vi "ReadMVC.vi"(9 "Max Time (s)":dbl=10.0, 11 "MVC Path":path) -> (1 "MVCpos":i32[](array[numeric]), 2 "MVCvalue":dbl[](array[numeric]), 3 "Muscles":string[](array[string]))   [LabVIEW 2015]
uses:
  EMG/EMG.lvclass
panel:
  out "Waveform Graph":dbl[][](graph)
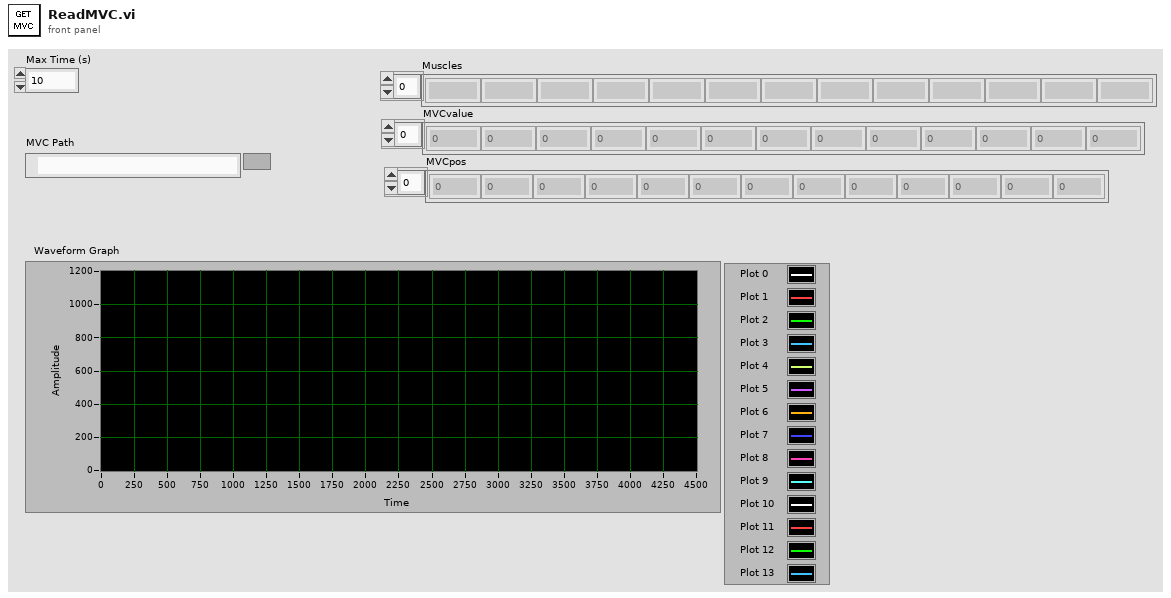
[diagram p1: front panel]
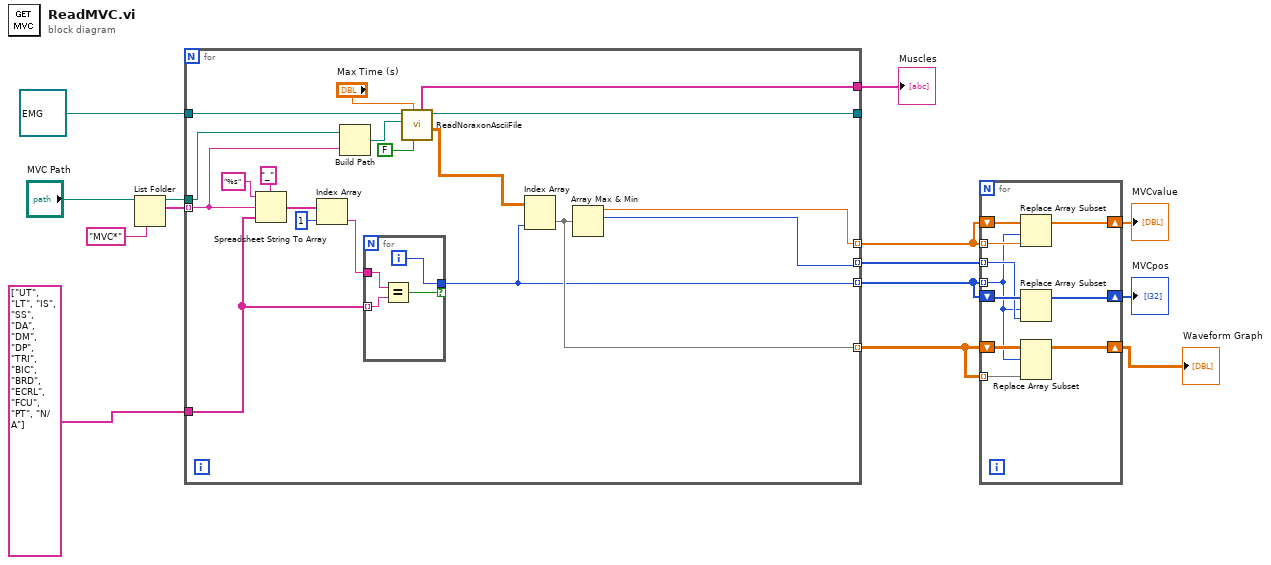
[diagram p0: block diagram]
diagram:
  n1 = List Folder(path="MVC Path", pattern="MVC*") -> (path out=w11:path, filenames=w12:string[])  [unwired: 2 in, 2 out]
  n2 = for {
    tunnel: w12 -> [w28] mode=indexing
    tunnel: w11 -> [w27]
    tunnel: string[] ["UT", "LT", "IS", "SS", "DA", "DM", "DP", "TRI", "BIC", "BRD", "ECRL", "FCU", "PT", "N/A"] -> [w26]
    tunnel: refnum<class "EMG.lvclass"> refnum ("EMG.lvclass") -> [w30]
    tunnel: [w24] -> _
    tunnel: [w15] -> w1
    tunnel: [w23] -> w4 mode=indexing
    tunnel: [w22] -> w8 mode=indexing
    tunnel: [w17] -> w5 mode=indexing
    tunnel: [w20] -> w2 mode=indexing
    n3 = Spreadsheet String To Array(delimiter (Tab)="_", format string="%s", spreadsheet string=w28, array type (2D Dbl)=w26) -> (array=w32:string[])
    n4 = Index Array(array=w32, index=1) -> (element=w25:string)
    n5 = Build Path(base path=w27, name or relative path=w28) -> (appended path=w29:path)
    n6 = for {
      tunnel: w26 -> [w37] mode=indexing
      tunnel: w25 -> [w36]
      tunnel: [w35] -> w17 if=w34
      i -> [w35]
      n7 = Equal?(x=w36, y=w37) -> (x = y?=w34:bool)
    }
    n8 = call "ReadNoraxonAsciiFile.vi"("With Sync (T)"=FALSE, "Max Time"="Max Time (s)", "Path"=w29, "EMG in"=w30) -> ("EMG"=w18:dbl[][], "EMG out"=w24:refnum<class "EMG.lvclass">, "Muscles"=w15:string[])  [unwired: 3 in, 2 out]
    n9 = Index Array(array=w18, index (col)=w17) -> (element=w20:dbl[])  [unwired: 1 in]
    n10 = Array Max & Min(array=w20) -> (max value=w23:dbl, max index (indices)=w22:i32)  [unwired: 2 out]
  }
  "Muscles" <- w1
  n11 = for {
    tunnel: w5 -> [w38] mode=indexing
    tunnel: w4 -> [w46] mode=indexing
    tunnel: w8 -> [w39] mode=indexing
    shift-right: [w44] -> w7
    shift-left: w4 -> [w47]
    shift-right: [w43] -> w6
    shift-left: w5 -> [w45]
    tunnel: w2 -> [w40] mode=indexing
    shift-right: [w42] -> w3
    shift-left: w2 -> [w41]
    n12 = Replace Array Subset(array=w47, new element=w46, index=w38) -> (w44:dbl[])
    n13 = Replace Array Subset(array=w45, new element=w39, index=w38) -> (w43:i32[])
    n14 = Replace Array Subset(array=w41, new element=w40, index (row)=w38) -> (w42:dbl[][])  [unwired: 1 in]
  }
  "MVCvalue" <- w7
  "MVCpos" <- w6
  "Waveform Graph" <- w3
